vi "FTW-SQLite-Core-QueryDebug.vi"(0 "SQL Script":string, 5 "Begin Timestamp":dbl format="%.3fmsec\n%<%D:%H:%M:%S%3u>t", 7 "Compile Time":dbl format="%.4psec", 9 "Rows Affected":i32=-1, 11 "error in":errorcluster) -> (4 "SQL Debug String":string, 15 "error out":errorcluster)   [LabVIEW 2014]
panel:
  # "Inputs"
  # "Outputs"
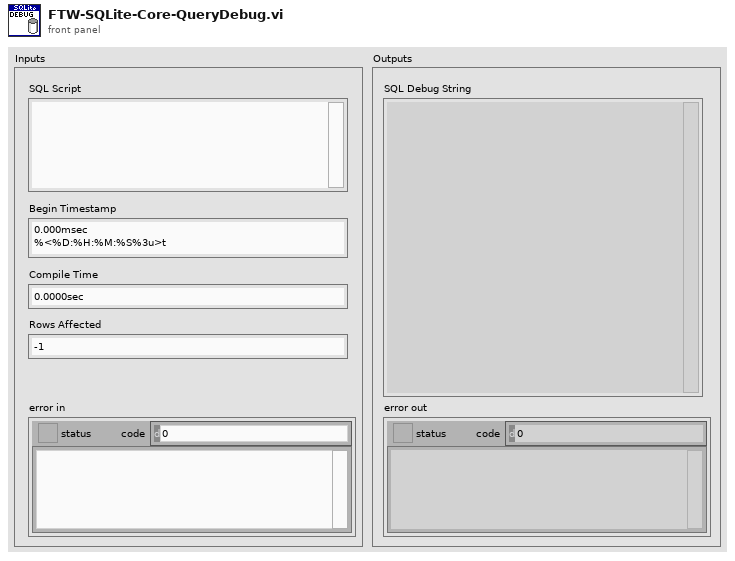
[diagram p1: front panel]
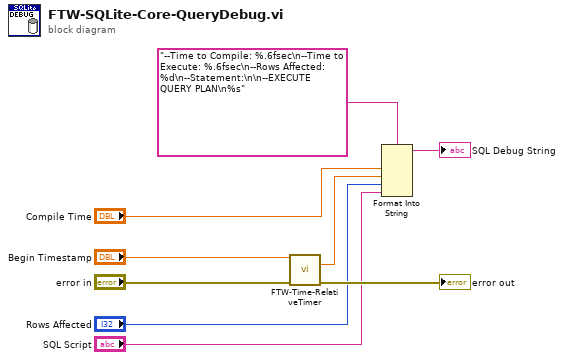
[diagram p0: block diagram]
diagram:
  n1 = call "FTW-Time-RelativeTimer.vi"("Previous Time"="Begin Timestamp", "error in"="error in") -> ("Elapsed Time"=w7:dbl, "error out"=→"error out":errorcluster)  [unwired: 11 in, 1 out]
  n2 = Format Into String(format string="--Time to Compile: %.6fsec\n--Time to Execute: %.6fsec\n--Rows Affected:   %d\n--Statement:\n\n--EXECUTE QUERY PLAN\n%s", "Compile Time", w7, "Rows Affected", "SQL Script") -> (resulting string=→"SQL Debug String":string)  [unwired: 2 in, 1 out]
